vi "setADCOffsetSensitivity.vi"(0 "ILCCommunications in":refnum<class "ILCCommunications.lvclass">, 1 "ILC in":refnum<class "ILC.lvclass">, 2 "Modbus in":refnum<class "IModbus.lvclass">, 3 "WaitForTrigger":bool, 4 "TriggerIRQ":bool, 5 "error in (no error)":errorcluster) -> (14 "ILCCommunications out":refnum<class "ILCCommunications.lvclass">, 15 "ILC out":refnum<class "ILC.lvclass">, 16 "Modbus out":refnum<class "IModbus.lvclass">, 19 "error out":errorcluster)   [LabVIEW 2016, in "ILCCommunications.lvclass"]
uses:
  ILCCommunications.lvclass
  Common_RT_ILC/ILC/ILC.lvclass
  Common_RT_Modbus/IModbus/IModbus.lvclass
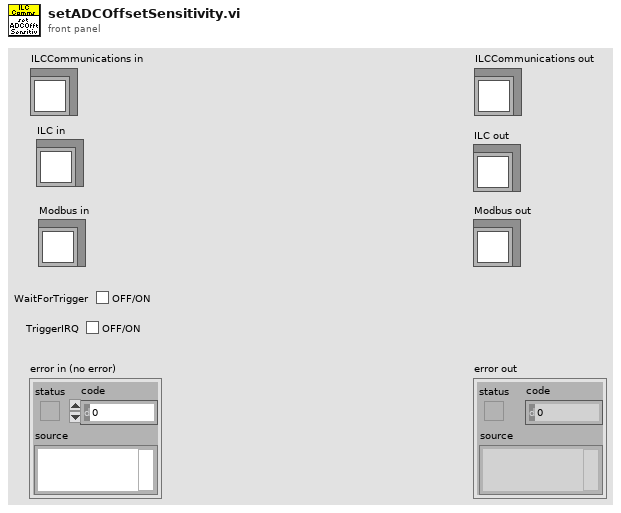
[diagram p1: front panel]
types:
  T1 = typedef "RTModbus.lvlib/TxFrame.ctl" = cluster{"Data":u8[], "WaitForTrigger":bool, "WaitForRx":u32, "TriggerIRQ":bool, "DelayMicroseconds":u16, "DelayMilliseconds":u16, "Timestamp":bool}
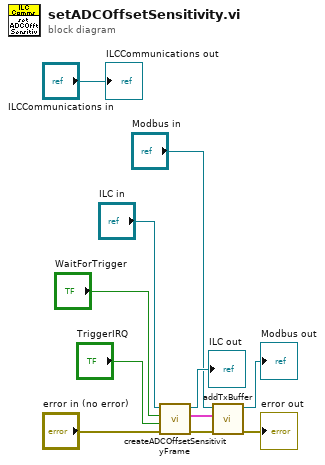
[diagram p0: block diagram]
diagram:
  n1 = call "createADCOffsetSensitivityFrame.vi"("error in (no error)"="error in (no error)", "TriggerIRQ"="TriggerIRQ", "WaitForTrigger"="WaitForTrigger", "ILC in"="ILC in") -> ("error out"=w8:errorcluster, "TxFrame"=w9:T1, "ILC out"=→"ILC out":refnum<class "ILC.lvclass">)  [unwired: 5 in]
  n2 = call-dynamic "addTxBuffer.vi"("error in (no error)"=w8, "TxFrame"=w9, "IModbus in"="Modbus in") -> ("error out"=→"error out":errorcluster, "IModbus out"=→"Modbus out":refnum<class "IModbus.lvclass">)  [unwired: 7 in]
  "ILCCommunications out" <- "ILCCommunications in"
